vi "Acquire.vi"(8 "error in (no error)":errorcluster, 10 "Msg in":T1, 11 "PXIDigitizer in":refnum<class "DaqPad_NI6009.lvclass">) -> (0 "error out":errorcluster, 1 "new command":string, 2 "Msg out":T1, 3 "PXIDigitizer out":refnum<class "DaqPad_NI6009.lvclass">)   [LabVIEW 2011, in "DaqPad_NI6009.lvclass"]
uses:
  DaqPad_NI6009.lvclass
  DriverMsg.ctl
  DaqPad_NI6009.lvclass/DaqPad_NI6009.ctl
  OnOffTypeDef.ctl
  DAQmx Fill In Error Info.vi
  BaseDriver/BaseDriver.lvclass
  C:/Program Files/National Instruments/LabVIEW 2011/resource/objmgr/daqmx.rc
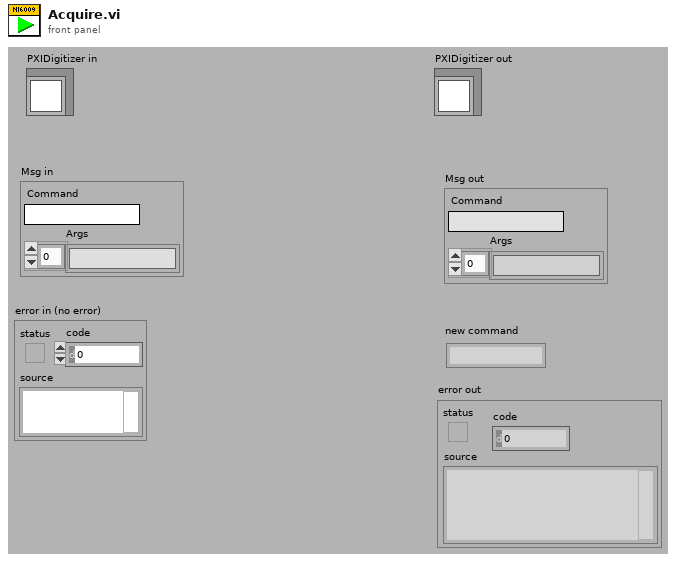
[diagram p1: front panel]
types:
  T1 = typedef "DriverMsg.ctl" = cluster{"Command":string, "Args":string[]}
  T2 = typedef "OnOffTypeDef.ctl" = enum16{"off", "on"}
  T3 = cluster{"Channel 0":dbl[], "Channel 1":dbl[], "Channel 2":dbl[], "Channel 3":dbl[]}
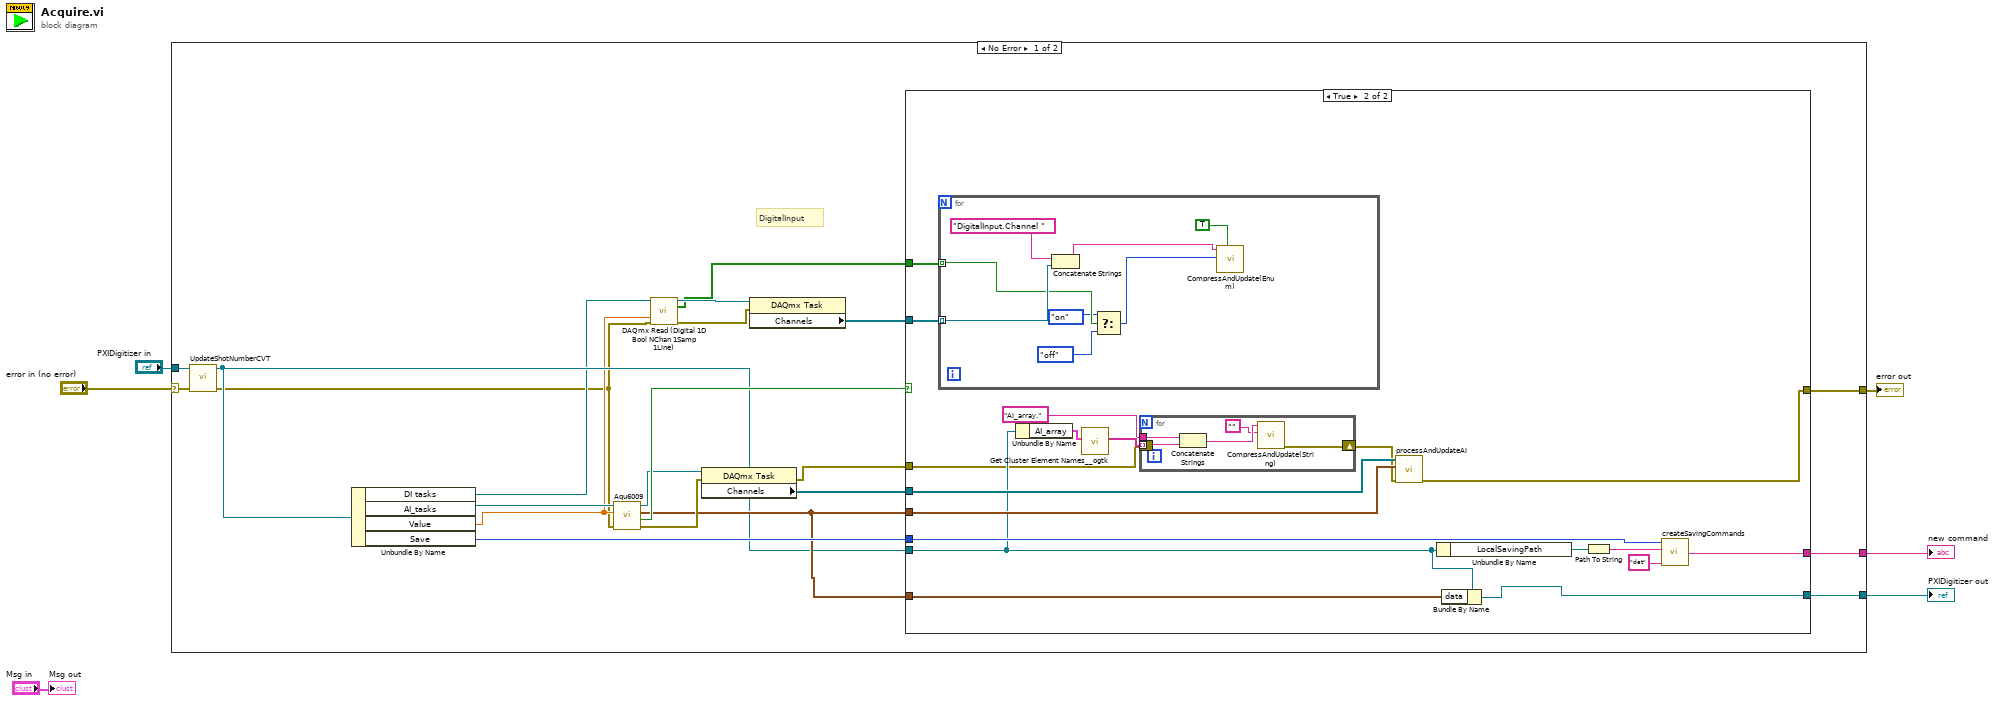
[diagram p0: block diagram]
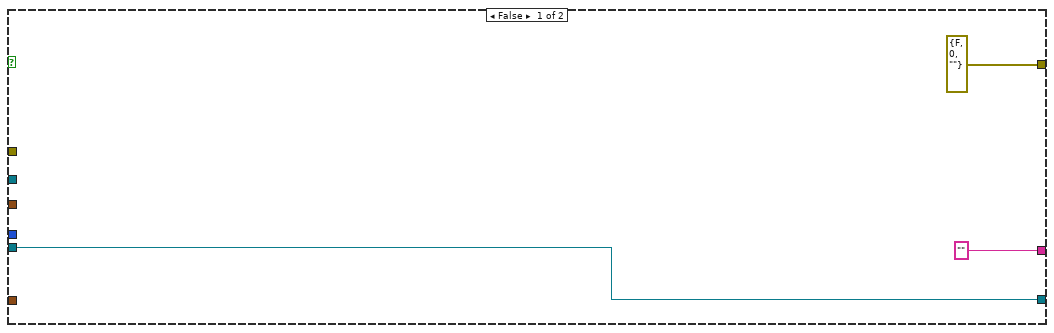
[diagram p2: hidden frame]
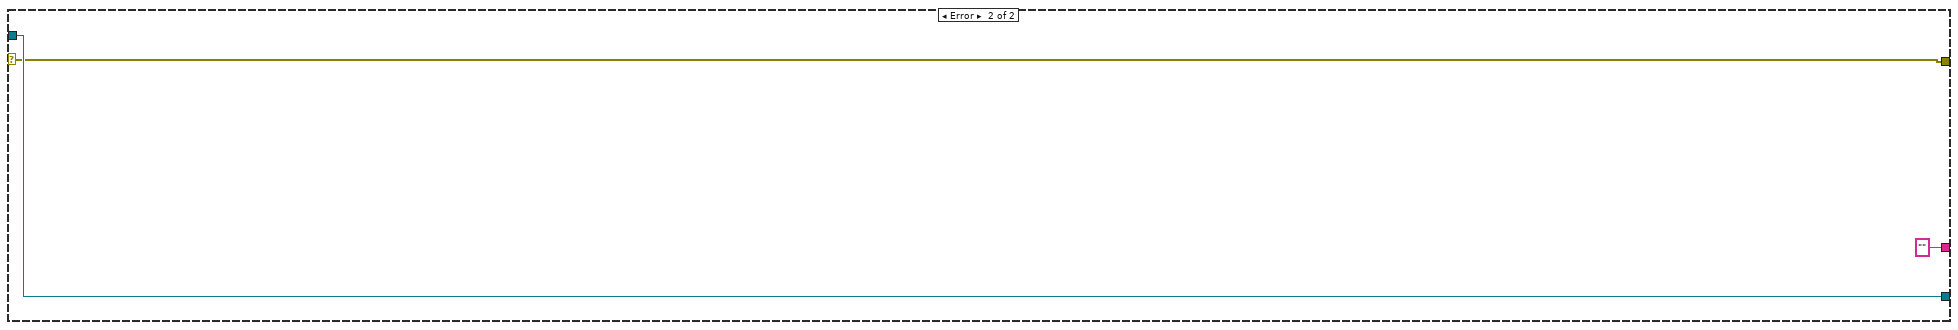
[diagram p3: hidden frame]
diagram:
  n1 = case shown="No Error" "error in (no error)" {
    selector: "error in (no error)" -> [w26 w63]
    tunnel: "PXIDigitizer in" -> [w27 w64]
    tunnel: [w22 w64] -> w6
    tunnel: [w23 w63] -> w4
    tunnel: [w24 "" ("new command")] -> w1
    frame No Error {
      # "DigitalInput"
      n2 = call "UpdateShotNumberCVT.vi"("error in (no error)"=w26, "BaseDriver in"=w27) -> ("error out"=w11:errorcluster, "BaseDriver out"=w14:refnum<class "DaqPad_NI6009.lvclass">)  [unwired: 8 in]
      n3 = Unbundle By Name(w14) -> ("DI tasks"=w13:refnum<k21>, "AI_tasks"=w21:refnum<k21>, "Value"=w12:dbl, "Save"=w25:T2)
      n4 = call "Aqu6009.vi"("error in (no error)"=w11, "timeout"=w12, "Refnum in"=w21) -> ("error out"=w16:errorcluster, "OK"=w20:bool, "data 2"=w15:waveform(dbl)[], "Refnum out"=w19:refnum<k21>)  [unwired: 5 in]
      n5 = call "DAQmx Read (Digital 1D Bool NChan 1Samp 1Line).vi"("task/channels in"=w13, "timeout"=w12, "error in"=w11) -> ("task out"=w10:refnum<k21>, "data"=w8:bool[], "error out"=w9:errorcluster)  [unwired: 10 in]
      n6 = property class="DAQmx Task"(reference=w19, error in=w16) -> (error out=w17:errorcluster, "Channels"=w18:refnum<k21>[])  [unwired: 1 out]
      n7 = property class="DAQmx Task"(reference=w10, error in=w9) -> ("Channels"=w7:refnum<k21>[])  [unwired: 2 out]
      n8 = case shown="True" w20 {
        tunnel: w25 -> [_ w48]
        tunnel: w14 -> [w28 w36]
        tunnel: ["" ("String") w44] -> w24
        tunnel: [errorcluster {"status"=FALSE, "code"=0, "source"=""} ("error IO") w42] -> w23
        tunnel: [w28 w39] -> w22
        tunnel: w15 -> [_ w41]
        tunnel: w18 -> [_ w43]
        tunnel: w17 -> [_ w32]
        tunnel: w15 -> [_ w40]
        tunnel: w8 -> [_ w37]
        tunnel: w7 -> [_ w38]
        frame False {
        }
        frame True {
          n9 = for {
            tunnel: w38 -> [w60] mode=indexing
            tunnel: w37 -> [w57] mode=indexing
            n10 = Concatenate Strings("DigitalInput.Channel " ("string"), w60) -> (w59:string)
            n11 = Select(t=OnOffTypeDef."on" ("Channel 0"), s=w57, f=OnOffTypeDef."off" ("Channel 0")) -> (s? t:f=w54:T2)
            n12 = call "CompressAndUpdate(Enum).vi"("force CVT update (false)"=TRUE, "enum variant"=w54, "command or variable name"=w59) -> ()  [unwired: 8 in, 1 out]
          }
          n13 = Unbundle By Name(w36) -> ("AI_array"=w35:T3)
          n14 = call "Get Cluster Element Names__ogtk.vi"("Cluster"=w35) -> ("Element Names"=w34:string[])  [unwired: 9 in, 1 out]
          n15 = for {
            tunnel: w34 -> [w53] mode=indexing
            tunnel: "Ai_array." ("string") -> [w52]
            shift-right: [w49] -> w31
            shift-left: w32 -> [_]
            n16 = Concatenate Strings(w52, w53) -> (w51:string)
            n17 = call "CompressAndUpdate(String).vi"("String"="", "command or variable name"=w51) -> ("error out"=w49:errorcluster)  [unwired: 9 in]
          }
          n18 = call "processAndUpdateAI.vi"("error in (no error)"=w31, "data in"=w41, "Channels"=w43) -> ("error out"=w42:errorcluster)  [unwired: 8 in]
          n19 = Unbundle By Name(w36) -> ("LocalSavingPath"=w45:path)
          n20 = Bundle By Name(cluster=w36, "data"=w40) -> (w39:refnum<class "DaqPad_NI6009.lvclass">)
          n21 = Path To String(path=w45) -> (string=w46:string)
          n22 = call "createSavingCommands.vi"("extension"="dat" ("Fileextension"), "Saving Path (local)"=w46, "Save"=w48) -> ("String"=w44:string)  [unwired: 1 in]
        }
      }
    }
    frame Error {
    }
  }
  "PXIDigitizer out" <- w6
  "error out" <- w4
  "new command" <- w1
  "Msg out" <- "Msg in"
